vi "SourceMirrorTrans.vi"(10 "EndPos":dbl, 11 "CurrPos":dbl) -> (2 "Curr Pos":dbl)   [LabVIEW 2015]
uses:
  Master Control 3_7 Folder/TMC/Set Parameter.ctl
  Master Control 3_7 Folder/LabView VI's/Source Mirror Manipulator/Axis.ctl
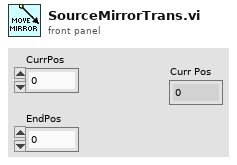
[diagram p1: front panel]
types:
  T1 = typedef "Axis.ctl" = enum16{"Translation", "Rotation"}
  T2 = typedef "Set Parameter.ctl" = enum16{"Acceleration (A)", "Baud Rate (BD)", "Counter 1 (C1)", "Counter 2 (C2)", "Control C Software Reset (CE)", "Check Sum Enable (CK)", "Clock Mode (CM)", "Clock Mode Ratio (CR)", "Clock Mode Out Step Width (CW)", "Deceleration (D)", "Digital Filtering, Input 1 (D1)", "Digital Filtering, Input 2 (D2)", "Digital Filtering, Input 3 (D3)", "Digital Filtering, Input 4 (D4)", "Digital Filtering, Input 5 (D5)", "Digital Filtering, Input 9 (D9)", "Digital Filtering, Input 10 (D10)", "Digital Filtering, Input 11 (D11)", "Digital Filtering, Input 12 (D12)", "Deadband (DB)", "Decrement Variable (DC)", "Enable/Disable Drive (DE)", "Device Name (DN)", "End Program Execution (E)", "Encoder Function Enable (EE)", "Encoder Lines (EL)", "Echo Mode (EM)", "Escape (ES)", "Execute Program at Address (EX)", "Hold (H)", "Hold Current (HC)", "Hold Current Delay Time (HI)", "Home to Encoder Index (HM)", "Home to Home Switch (HT)", "Increment Variable (IC)", "Initialize Parameters to NVM (IP)", "Input into Variable (IV)", "Jog Enable (JE)", "Limit Stop Mode (LM)", "Move Absolute (MA)", "Move Relative (MR)", "MicroStepping Select (MS)", "Motor Settling Delay Time (MT)", "Output 1 (O1)", "Output 2 (O2)", "Output 3 (O3)", "Output 4 (O4)", "Output 9 (O9)", "Output 10 (O10)", "Output 11 (O11)", "Output 12 (O12)", "Output High Byte (9-12) (OH)", "Output Low Byte (1-4) (OL)", "Output Total (1-4 and 9-12) (OT)", "Position Maintenance (PM)", "Party Mode (PY)", "Register 1 (R1)", "Register 2 (R2)", "Register 3 (R3)", "Register 4 (R4)", "Run Current (RC)", "Stall Factor (SF)", "Slew (SL)", "Stall Mode Set (SM)", "Upgrade Firmware (UG)", "Velocity Initial (VI)", "Velocity Maximum (VM)"}
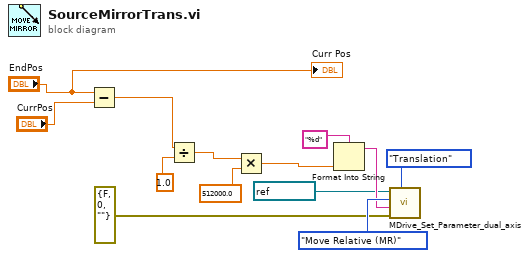
[diagram p0: block diagram]
diagram:
  n1 = Subtract(x="EndPos", y="CurrPos") -> (x-y=w2:dbl)
  n2 = Divide(x=w2, y=1.0) -> (x/y=w5:dbl)
  n3 = Multiply(x=w5, y=512000.0 ("x")) -> (x*y=w7:dbl)
  n4 = Format Into String(format string="%d", w7) -> (resulting string=w11:string)  [unwired: 2 in, 1 out]
  n5 = call "MDrive_Set_Parameter_dual_axis.vi"("Axis"=Axis."Translation", "error in"=errorcluster {"status"=FALSE, "code"=0, "source"=""} ("error constant"), "Parameter Setpoint"=w11, "Set Parameter"=Set_Parameter."Move Relative (MR)", "VISA resource name in"=refnum<visa-resource-name> "COM5" ("VISA resource name")) -> ()  [unwired: 2 in, 2 out]
  "Curr Pos" <- "EndPos"
